vi "SignalGenerator.vi"(9 "Amplitude":dbl, 10 "Frequency":dbl) -> (2 "error out":errorcluster)   [LabVIEW 2015]
panel:
  out "error in":errorcluster caption="error out"
  in  "Stop":bool
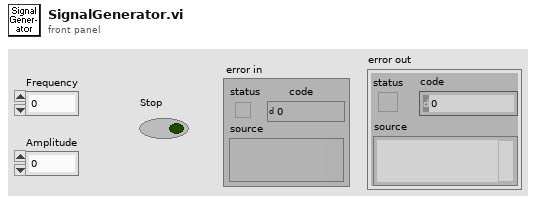
[diagram p1: front panel]
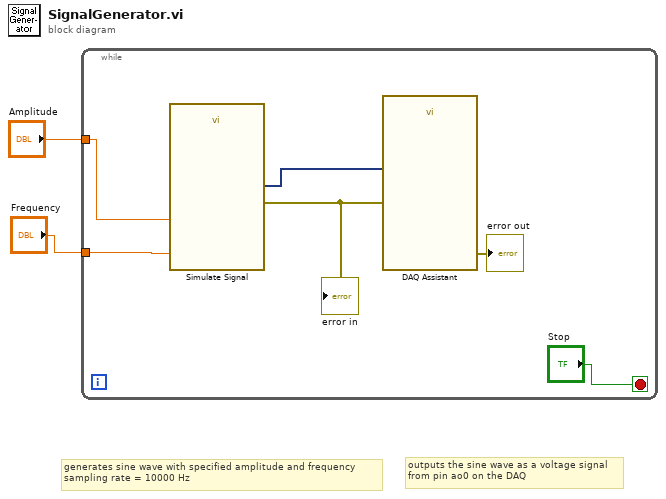
[diagram p0: block diagram]
diagram:
  # "outputs the sine wave as a voltage signal\nfrom pin ao0 on the DAQ"
  # "generates sine wave with specified amplitude and frequency\nsampling rate = 10000 Hz"
  n1 = while {
    tunnel: "Amplitude" -> [w3]
    tunnel: "Frequency" -> [w8]
    stop <- "Stop" stop-if-true
    n2 = call "Simulate Signal"("Frequency"=w8, "Amplitude"=w3) -> ("Sine"=w7:dynamicdata, "error out"=w6:errorcluster)  [unwired: 12 in]
    "error in" <- w6
    n3 = call "DAQ Assistant"("data"=w7, "error in"=w6) -> ("error out"=→"error out":errorcluster)  [unwired: 15 in, 2 out]
  }
